vi "G2CPU Line Fit.vi"(6 "Auto Release Coordinates In (Enabled)":T1={"Auto Release X Coordinates (Enabled)"=TRUE, "Auto Release Y Coordinates (Enabled)"=TRUE, "Auto Release Keys (Enabled)"=TRUE}, 8 "error in":errorcluster, 11 "Coordinates In":T3) -> (0 "error out":errorcluster, 3 "Fits Out":T2)   [LabVIEW 2020, in "G2CPU Line Profile.lvlib"]
doc: "Perform a linear fit on the image coordinates in order to find the best fit based on keys grouping.\nThe output value are defined as Ax + By + C = 0"
uses:
  G2CPU Line Profile.lvlib
  <vilib>/Natan Biesmans/G2CPU GPU and CPU HPC Toolkit/G2CPU Libraries/Arrays/1DArray/f32/1D Array f32.lvclass
  C:/Program Files/National Instruments/LabVIEW 2025/vi.lib/Natan Biesmans/G2CPU GPU and CPU HPC Toolkit/G2CPU Libraries/Arrays/Array/Array Prototype.lvclass
  <vilib>/Natan Biesmans/G2CPU GPU and CPU HPC Toolkit/G2CPU Libraries/Arrays/1DArray/u32/1D Array u32.lvclass
  <vilib>/Natan Biesmans/G2CPU GPU and CPU HPC Toolkit/G2CPU Libraries/Arrays/Array/Array Prototype.lvclass/Array Prototype.ctl
  39b00889-5bfe-4fc8-ae9c-3ebe22e068e1.vi
  e67f2f6d-116c-41ca-99d3-9b58d0d13c14.vi
  aad3cb97-5a1b-40f0-9ba0-792b29d533f0.vi
  d1bde40f-3aaf-4b83-8085-08b903dc0029.vi
  4a28855f-6dfd-4182-87fd-1eece1cf3a87.vi
  35915ded-74a9-4bdb-827f-ed8d931a8cd9.vi
  6dbd2c3f-d680-484a-89ae-c41d1444e36a.vi
  4433cce3-d785-4f34-afb2-5ec678587074.vi
  c524c46e-5266-4137-881e-03e53a651323.vi
  7ee46f17-b792-4bdf-bc78-f6f359ee11a0.vi
  685ef3a2-bc3e-421d-ae28-b6af0c72629d.vi
  1c28c6f9-52d4-4ee1-85fd-97d058665e62.vi
  c12179c3-812a-4d4b-9674-be382bedbea4.vi
  28c67a32-5845-438f-b6be-fac02040104b.vi
  e957327c-ca5c-4585-a2df-5463998674b4.vi
  <vilib>/Natan Biesmans/G2CPU GPU and CPU HPC Toolkit/G2CPU Libraries/Arrays/Array/G2CPU Get Array Pointer.vi
  39b00889-5bfe-4fc8-ae9c-3ebe22e068e1.vi/2cbae9c5-d993-4013-91e6-67de96abb5a0.vi
  39b00889-5bfe-4fc8-ae9c-3ebe22e068e1.vi/df7b902d-6356-419a-b5d5-2ac54df1e506.vi
  e67f2f6d-116c-41ca-99d3-9b58d0d13c14.vi/2cbae9c5-d993-4013-91e6-67de96abb5a0.vi
  e67f2f6d-116c-41ca-99d3-9b58d0d13c14.vi/df7b902d-6356-419a-b5d5-2ac54df1e506.vi
  aad3cb97-5a1b-40f0-9ba0-792b29d533f0.vi/bd8c0049-2ad4-4080-93a3-884a36f051e6.vi
  aad3cb97-5a1b-40f0-9ba0-792b29d533f0.vi/509954f5-3710-4f12-85e8-176e1832af7a.vi
  d1bde40f-3aaf-4b83-8085-08b903dc0029.vi/f4654d05-beb0-4753-bab7-24376daae318.vi
  d1bde40f-3aaf-4b83-8085-08b903dc0029.vi/a2f9e1c9-c94e-4cd6-9432-cf54c3ac582a.vi
  4a28855f-6dfd-4182-87fd-1eece1cf3a87.vi/a7ec311c-7cd8-4650-9526-d70ff0a769d1.vi
  35915ded-74a9-4bdb-827f-ed8d931a8cd9.vi/2e03f477-51b7-4ba0-bb4f-4f838f6557e6.vi
  35915ded-74a9-4bdb-827f-ed8d931a8cd9.vi/125d45d4-836b-469d-8a4a-6adb452f866d.vi
  35915ded-74a9-4bdb-827f-ed8d931a8cd9.vi/8038e9ed-2e71-4568-91ba-0d873494c5ed.vi
  6dbd2c3f-d680-484a-89ae-c41d1444e36a.vi/2e03f477-51b7-4ba0-bb4f-4f838f6557e6.vi
  6dbd2c3f-d680-484a-89ae-c41d1444e36a.vi/125d45d4-836b-469d-8a4a-6adb452f866d.vi
  6dbd2c3f-d680-484a-89ae-c41d1444e36a.vi/8038e9ed-2e71-4568-91ba-0d873494c5ed.vi
  4433cce3-d785-4f34-afb2-5ec678587074.vi/2e03f477-51b7-4ba0-bb4f-4f838f6557e6.vi
  4433cce3-d785-4f34-afb2-5ec678587074.vi/125d45d4-836b-469d-8a4a-6adb452f866d.vi
  4433cce3-d785-4f34-afb2-5ec678587074.vi/8038e9ed-2e71-4568-91ba-0d873494c5ed.vi
  c524c46e-5266-4137-881e-03e53a651323.vi/def40612-844c-421c-bb75-87c330777b0b.vi
  7ee46f17-b792-4bdf-bc78-f6f359ee11a0.vi/7c469f53-f2d9-4897-b214-93bda7c45308.vi
  7ee46f17-b792-4bdf-bc78-f6f359ee11a0.vi/f1659385-6fa7-48ef-9230-58e699f02080.vi
  685ef3a2-bc3e-421d-ae28-b6af0c72629d.vi/cfed8f62-9c64-4dab-912e-5e7c21cb720b.vi
  1c28c6f9-52d4-4ee1-85fd-97d058665e62.vi/d8f9d983-4edf-44a2-8364-f00f0b470774.vi
  1c28c6f9-52d4-4ee1-85fd-97d058665e62.vi/83167447-a0f5-45d9-a71d-4def8f50970d.vi
  c12179c3-812a-4d4b-9674-be382bedbea4.vi/cfed8f62-9c64-4dab-912e-5e7c21cb720b.vi
  28c67a32-5845-438f-b6be-fac02040104b.vi/d8f9d983-4edf-44a2-8364-f00f0b470774.vi
  28c67a32-5845-438f-b6be-fac02040104b.vi/83167447-a0f5-45d9-a71d-4def8f50970d.vi
  e957327c-ca5c-4585-a2df-5463998674b4.vi/d8f9d983-4edf-44a2-8364-f00f0b470774.vi
  e957327c-ca5c-4585-a2df-5463998674b4.vi/83167447-a0f5-45d9-a71d-4def8f50970d.vi
  39b00889-5bfe-4fc8-ae9c-3ebe22e068e1.vi/df7b902d-6356-419a-b5d5-2ac54df1e506.vi/6058dca8-195d-4566-b47b-6d6a1c5af61f.vi
  e67f2f6d-116c-41ca-99d3-9b58d0d13c14.vi/df7b902d-6356-419a-b5d5-2ac54df1e506.vi/6058dca8-195d-4566-b47b-6d6a1c5af61f.vi
  aad3cb97-5a1b-40f0-9ba0-792b29d533f0.vi/509954f5-3710-4f12-85e8-176e1832af7a.vi/edd31282-7992-4bba-af75-482693dee5e1.vi
  35915ded-74a9-4bdb-827f-ed8d931a8cd9.vi/2e03f477-51b7-4ba0-bb4f-4f838f6557e6.vi/d8e2d9cc-c923-495e-b121-b6b84788c73f.vi
  35915ded-74a9-4bdb-827f-ed8d931a8cd9.vi/2e03f477-51b7-4ba0-bb4f-4f838f6557e6.vi/345e91f0-9a5e-4de4-af9c-133346717e4a.vi
  6dbd2c3f-d680-484a-89ae-c41d1444e36a.vi/2e03f477-51b7-4ba0-bb4f-4f838f6557e6.vi/d8e2d9cc-c923-495e-b121-b6b84788c73f.vi
  6dbd2c3f-d680-484a-89ae-c41d1444e36a.vi/2e03f477-51b7-4ba0-bb4f-4f838f6557e6.vi/345e91f0-9a5e-4de4-af9c-133346717e4a.vi
  4433cce3-d785-4f34-afb2-5ec678587074.vi/2e03f477-51b7-4ba0-bb4f-4f838f6557e6.vi/d8e2d9cc-c923-495e-b121-b6b84788c73f.vi
  4433cce3-d785-4f34-afb2-5ec678587074.vi/2e03f477-51b7-4ba0-bb4f-4f838f6557e6.vi/345e91f0-9a5e-4de4-af9c-133346717e4a.vi
  7ee46f17-b792-4bdf-bc78-f6f359ee11a0.vi/7c469f53-f2d9-4897-b214-93bda7c45308.vi/6058dca8-195d-4566-b47b-6d6a1c5af61f.vi
  685ef3a2-bc3e-421d-ae28-b6af0c72629d.vi/cfed8f62-9c64-4dab-912e-5e7c21cb720b.vi/77c7badc-ed81-4514-99c1-20d37f4e5ecc.vi
  685ef3a2-bc3e-421d-ae28-b6af0c72629d.vi/cfed8f62-9c64-4dab-912e-5e7c21cb720b.vi/eb76fa01-6782-47b4-b34f-9eb474c9cc78.vi
  <vilib>/Natan Biesmans/G2CPU GPU and CPU HPC Toolkit/ArrayFire Driver/VIs/Run as Multi Device.vi
  c12179c3-812a-4d4b-9674-be382bedbea4.vi/cfed8f62-9c64-4dab-912e-5e7c21cb720b.vi/77c7badc-ed81-4514-99c1-20d37f4e5ecc.vi
  c12179c3-812a-4d4b-9674-be382bedbea4.vi/cfed8f62-9c64-4dab-912e-5e7c21cb720b.vi/eb76fa01-6782-47b4-b34f-9eb474c9cc78.vi
  39b00889-5bfe-4fc8-ae9c-3ebe22e068e1.vi/df7b902d-6356-419a-b5d5-2ac54df1e506.vi/6058dca8-195d-4566-b47b-6d6a1c5af61f.vi/77c7badc-ed81-4514-99c1-20d37f4e5ecc.vi
  39b00889-5bfe-4fc8-ae9c-3ebe22e068e1.vi/df7b902d-6356-419a-b5d5-2ac54df1e506.vi/6058dca8-195d-4566-b47b-6d6a1c5af61f.vi/eb76fa01-6782-47b4-b34f-9eb474c9cc78.vi
  e67f2f6d-116c-41ca-99d3-9b58d0d13c14.vi/df7b902d-6356-419a-b5d5-2ac54df1e506.vi/6058dca8-195d-4566-b47b-6d6a1c5af61f.vi/77c7badc-ed81-4514-99c1-20d37f4e5ecc.vi
  e67f2f6d-116c-41ca-99d3-9b58d0d13c14.vi/df7b902d-6356-419a-b5d5-2ac54df1e506.vi/6058dca8-195d-4566-b47b-6d6a1c5af61f.vi/eb76fa01-6782-47b4-b34f-9eb474c9cc78.vi
  7ee46f17-b792-4bdf-bc78-f6f359ee11a0.vi/7c469f53-f2d9-4897-b214-93bda7c45308.vi/6058dca8-195d-4566-b47b-6d6a1c5af61f.vi/77c7badc-ed81-4514-99c1-20d37f4e5ecc.vi
  7ee46f17-b792-4bdf-bc78-f6f359ee11a0.vi/7c469f53-f2d9-4897-b214-93bda7c45308.vi/6058dca8-195d-4566-b47b-6d6a1c5af61f.vi/eb76fa01-6782-47b4-b34f-9eb474c9cc78.vi
  <vilib>/Natan Biesmans/G2CPU GPU and CPU HPC Toolkit/G2CPU Libraries/Arrays/1DArray/binary/1D Array binary.lvclass
  <vilib>/Natan Biesmans/G2CPU GPU and CPU HPC Toolkit/G2CPU Libraries/Arrays/1DArray/s32/1D Array s32.lvclass
  <vilib>/Natan Biesmans/G2CPU GPU and CPU HPC Toolkit/ArrayFire Driver/VIs/iszero.vi
  <vilib>/Natan Biesmans/G2CPU GPU and CPU HPC Toolkit/ArrayFire Driver/VIs/sub.vi
  <vilib>/Natan Biesmans/G2CPU GPU and CPU HPC Toolkit/ArrayFire Driver/VIs/release array.vi
  <vilib>/Natan Biesmans/G2CPU GPU and CPU HPC Toolkit/ArrayFire Driver/subvi/Error Converter (ErrCode or Status).vi
  <vilib>/Natan Biesmans/G2CPU GPU and CPU HPC Toolkit/ArrayFire Driver/VIs/cast.vi
  <vilib>/Natan Biesmans/G2CPU GPU and CPU HPC Toolkit/ArrayFire Driver/VIs/add.vi
  <vilib>/Natan Biesmans/G2CPU GPU and CPU HPC Toolkit/G2CPU Libraries/Arrays/Array/G2CPU Set Array Pointer.vi
  <vilib>/Natan Biesmans/G2CPU GPU and CPU HPC Toolkit/ArrayFire Driver/VIs/lt.vi
  <vilib>/Natan Biesmans/G2CPU GPU and CPU HPC Toolkit/ArrayFire Driver/VIs/or.vi
  <vilib>/Natan Biesmans/G2CPU GPU and CPU HPC Toolkit/ArrayFire Driver/VIs/not.vi
  <vilib>/Natan Biesmans/G2CPU GPU and CPU HPC Toolkit/ArrayFire Driver/VIs/where.vi
  <vilib>/Natan Biesmans/G2CPU GPU and CPU HPC Toolkit/ArrayFire Driver/VIs/lookup.vi
  <vilib>/Natan Biesmans/G2CPU GPU and CPU HPC Toolkit/ArrayFire Driver/VIs/abs.vi
  <vilib>/Natan Biesmans/G2CPU GPU and CPU HPC Toolkit/ArrayFire Driver/VIs/le.vi
  <vilib>/Natan Biesmans/G2CPU GPU and CPU HPC Toolkit/ArrayFire Driver/VIs/replace.vi
  <vilib>/Natan Biesmans/G2CPU GPU and CPU HPC Toolkit/G2CPU Libraries/Arrays/Array/Array Prototype.lvclass
  <vilib>/Natan Biesmans/G2CPU GPU and CPU HPC Toolkit/G2CPU Libraries/Arrays/1DArray/1D Array Prototype.lvclass
  <vilib>/Natan Biesmans/G2CPU GPU and CPU HPC Toolkit/G2CPU Libraries/Arrays/DataTypes/I32/s32.lvclass
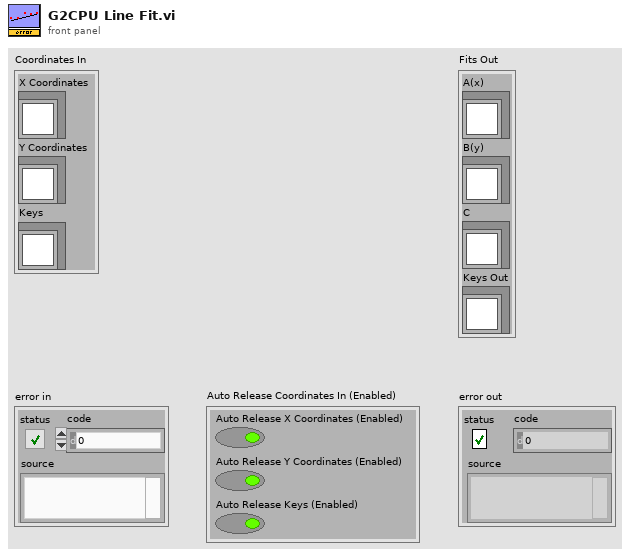
[diagram p1: front panel]
types:
  T1 = cluster{"Auto Release X Coordinates (Enabled)":bool, "Auto Release Y Coordinates (Enabled)":bool, "Auto Release Keys (Enabled)":bool}
  T2 = cluster{"A(x)":refnum<class "1D Array f32.lvclass">, "B(y)":refnum<class "1D Array f32.lvclass">, "C":refnum<class "1D Array f32.lvclass">, "Keys Out":refnum<class "1D Array u32.lvclass">}
  T3 = cluster{"X Coordinates":refnum<class "1D Array f32.lvclass">, "Y Coordinates":refnum<class "1D Array f32.lvclass">, "Keys":refnum<class "1D Array u32.lvclass">}
  T4 = cluster{"A":refnum<class "1D Array f32.lvclass">, "B":refnum<class "1D Array f32.lvclass">, "C":refnum<class "1D Array f32.lvclass">, "Keys Out":refnum<class "1D Array u32.lvclass">}
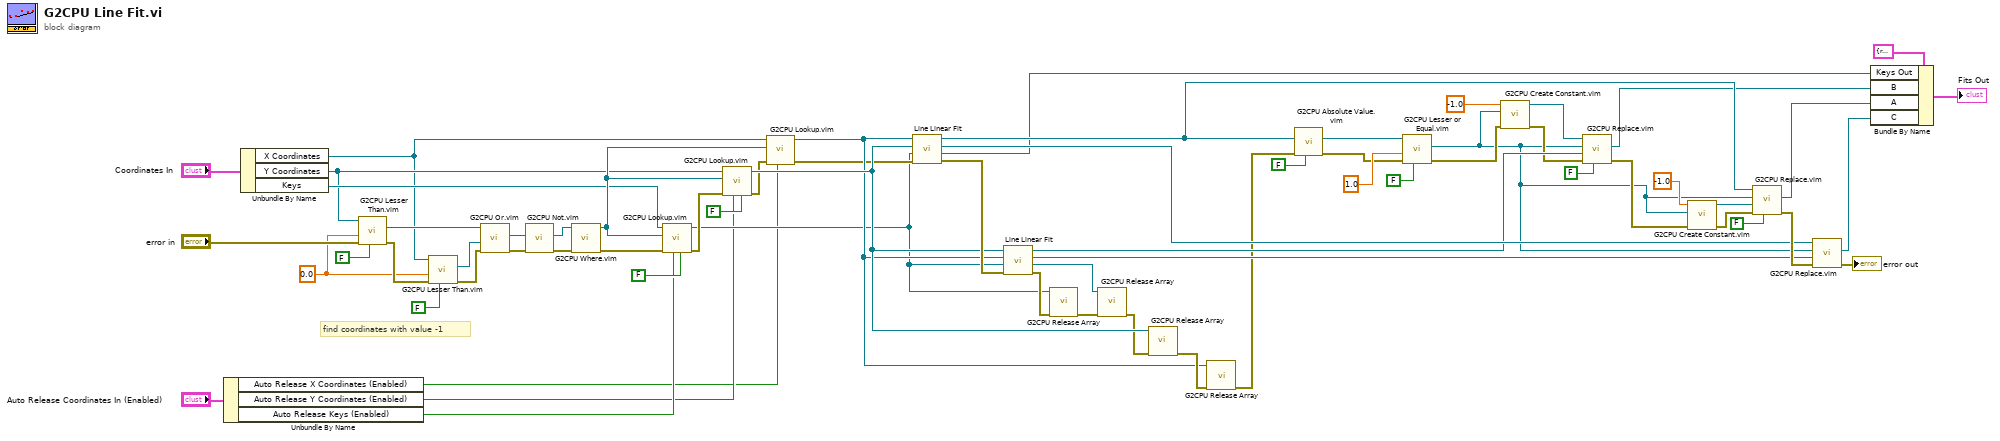
[diagram p0: block diagram]
diagram:
  w26 = sgl 0.0
  # "find coordinates with value -1"
  n1 = Unbundle By Name("Auto Release Coordinates In (Enabled)") -> ("Auto Release X Coordinates (Enabled)"=w1:bool, "Auto Release Y Coordinates (Enabled)"=w2:bool, "Auto Release Keys (Enabled)"=w3:bool)
  n2 = Unbundle By Name("Coordinates In") -> ("X Coordinates"=w11:refnum<class "1D Array f32.lvclass">, "Y Coordinates"=w12:refnum<class "1D Array f32.lvclass">, "Keys"=w13:refnum<class "1D Array u32.lvclass">)
  n3 = call "G2CPU Lesser Than.vim"("Auto Release lhs (Enabled)"=FALSE ("Auto Release rhs (Enabled)"), "error in (no error)"="error in", "Array rhs"=w26, "Array lhs"=w12) -> ("error out"=w39:errorcluster, "Array Result"=w37:refnum<class "1D Array binary.lvclass">)  [unwired: 6 in]
  n4 = call "G2CPU Lesser Than.vim"("Auto Release lhs (Enabled)"=FALSE ("Auto Release rhs (Enabled)"), "error in (no error)"=w39, "Array rhs"=w26, "Array lhs"=w11) -> ("error out"=w36:errorcluster, "Array Result"=w38:refnum<class "1D Array binary.lvclass">)  [unwired: 6 in]
  n5 = call "G2CPU Or.vim"("error in (no error)"=w36, "Array rhs"=w38, "Array lhs"=w37) -> ("error out"=w35:errorcluster, "Array Result"=w34:refnum<class "1D Array binary.lvclass">)  [unwired: 7 in]
  n6 = call "G2CPU Not.vim"("error in (no error)"=w35, "Array in"=w34) -> ("error out"=w33:errorcluster, "Array Result"=w32:refnum<class "1D Array binary.lvclass">)  [unwired: 8 in]
  n7 = call "G2CPU Where.vim"("error in (no error)"=w33, "Array in"=w32) -> ("error out"=w19:errorcluster, "Non Zero Indices"=w17:refnum<class "1D Array u32.lvclass">)  [unwired: 8 in]
  n8 = call "G2CPU Lookup.vim"("Auto Release Indices (Enabled)"=FALSE, "Auto Release Array In (Enabled)"=w3, "error in (no error)"=w19, "Indices (1D)"=w17, "Array In"=w13) -> ("error out"=w18:errorcluster, "Indexed Array"=w16:refnum<class "1D Array u32.lvclass">)  [unwired: 5 in]
  n9 = call "G2CPU Lookup.vim"("Auto Release Indices (Enabled)"=FALSE, "Auto Release Array In (Enabled)"=w2, "error in (no error)"=w18, "Indices (1D)"=w17, "Array In"=w12) -> ("error out"=w29:errorcluster, "Indexed Array"=w31:refnum<class "1D Array f32.lvclass">)  [unwired: 5 in]
  n10 = call "G2CPU Lookup.vim"("Auto Release Array In (Enabled)"=w1, "error in (no error)"=w29, "Indices (1D)"=w17, "Array In"=w11) -> ("error out"=w28:errorcluster, "Indexed Array"=w30:refnum<class "1D Array f32.lvclass">)  [unwired: 6 in]
  n11 = call "Line Linear Fit.vi"("error in"=w28, "Keys"=w16, "Y"=w31, "X"=w30) -> ("error out"=w65:errorcluster, "Keys"=w5:refnum<class "1D Array u32.lvclass">, "Offset"=w58:refnum<class "1D Array f32.lvclass">, "Slope"=w56:refnum<class "1D Array f32.lvclass">)  [unwired: 4 in]
  n12 = call "Line Linear Fit.vi"("error in"=w65, "Keys"=w16, "Y"=w30, "X"=w31) -> ("error out"=w23:errorcluster, "Keys"=w20:refnum<class "1D Array u32.lvclass">, "Offset"=w59:refnum<class "1D Array f32.lvclass">, "Slope"=w57:refnum<class "1D Array f32.lvclass">)  [unwired: 4 in]
  n13 = call <vilib>:"G2CPU Release Array.vi"("error in (no error)"=w23, "Array in"=w16) -> ("error out"=w22:errorcluster)  [unwired: 9 in]
  n14 = call <vilib>:"G2CPU Release Array.vi"("error in (no error)"=w22, "Array in"=w20) -> ("error out"=w21:errorcluster)  [unwired: 9 in]
  n15 = call <vilib>:"G2CPU Release Array.vi"("error in (no error)"=w21, "Array in"=w31) -> ("error out"=w64:errorcluster)  [unwired: 9 in]
  n16 = call <vilib>:"G2CPU Release Array.vi"("error in (no error)"=w64, "Array in"=w30) -> ("error out"=w55:errorcluster)  [unwired: 9 in]
  n17 = call "G2CPU Absolute Value.vim"("Auto Release (Enabled)"=FALSE, "error in (no error)"=w55, "Array in"=w56) -> ("error out"=w53:errorcluster, "Array Result"=w54:refnum<class "1D Array f32.lvclass">)  [unwired: 7 in]
  n18 = call "G2CPU Lesser or Equal.vim"("Auto Release lhs (Enabled)"=FALSE, "error in (no error)"=w53, "Array rhs"=sgl 1.0, "Array lhs"=w54) -> ("error out"=w50:errorcluster, "Array Result"=w46:refnum<class "1D Array binary.lvclass">)  [unwired: 6 in]
  n19 = call "G2CPU Create Constant.vim"("error in (no error)"=w50, "Size"=w46, "val"=sgl -1.0) -> ("error out"=w49:errorcluster, "object out"=w51:refnum<class "1D Array f32.lvclass">)  [unwired: 7 in]
  n20 = call "G2CPU Replace.vim"("Auto Release Replace Condition (Enabled)"=FALSE, "error in (no error)"=w49, "To Replace Values Array or scalar Value"=w57, "Replace  Condition"=w46, "Array In"=w51) -> ("error out"=w47:errorcluster, "Array out (same as in)"=w6:refnum<class "1D Array f32.lvclass">)  [unwired: 5 in]
  n21 = call "G2CPU Create Constant.vim"("error in (no error)"=w47, "Size"=w46, "val"=sgl -1.0) -> ("error out"=w44:errorcluster, "object out"=w45:refnum<class "1D Array f32.lvclass">)  [unwired: 7 in]
  n22 = call "G2CPU Replace.vim"("Auto Release Replace Condition (Enabled)"=FALSE, "error in (no error)"=w44, "To Replace Values Array or scalar Value"=w45, "Replace  Condition"=w46, "Array In"=w56) -> ("error out"=w61:errorcluster, "Array out (same as in)"=w7:refnum<class "1D Array f32.lvclass">)  [unwired: 5 in]
  n23 = call "G2CPU Replace.vim"("error in (no error)"=w61, "To Replace Values Array or scalar Value"=w59, "Replace  Condition"=w46, "Array In"=w58) -> ("error out"=→"error out":errorcluster, "Array out (same as in)"=w8:refnum<class "1D Array f32.lvclass">)  [unwired: 6 in]
  n24 = Bundle By Name(cluster=T4 {"A"=refnum, "B"=refnum, "C"=refnum, "Keys Out"=refnum} ("Cluster"), "Keys Out"=w5, "B"=w6, "A"=w7, "C"=w8) -> (→"Fits Out":T4)
